vi "DBL Pointer.Set Channel Count.vi"(10 "channel count":u64, 11 "DBL Buffer in":refnum<class "DBL Pointer.lvclass">) -> (3 "DBL Buffer out":refnum<class "DBL Pointer.lvclass">)   [LabVIEW 2017, in "DSF.Engine.lvlib" / "DBL Pointer.lvclass"]
uses:
  DBL Pointer.lvclass
  DBL Pointer.lvclass/DBL Pointer.ctl
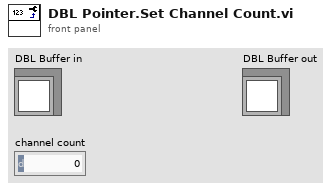
[diagram p1: front panel]
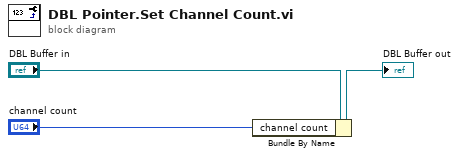
[diagram p0: block diagram]
diagram:
  n1 = Bundle By Name(cluster="DBL Buffer in", "channel count"="channel count") -> (→"DBL Buffer out":refnum<class "DBL Pointer.lvclass">)
